vi "Write handle.vi"(8 "error in (no error)":errorcluster, 10 "handle":u64, 11 "Synnax Writer in":refnum<class "Synnax Writer.lvclass">) -> (0 "error out":errorcluster, 3 "Synnax Writer out":refnum<class "Synnax Writer.lvclass">)   [LabVIEW 2026, in "synnax_clib.lvlib" / "Synnax Writer.lvclass"]
uses:
  Synnax Writer.lvclass
  Synnax Writer.lvclass/Synnax Writer.ctl
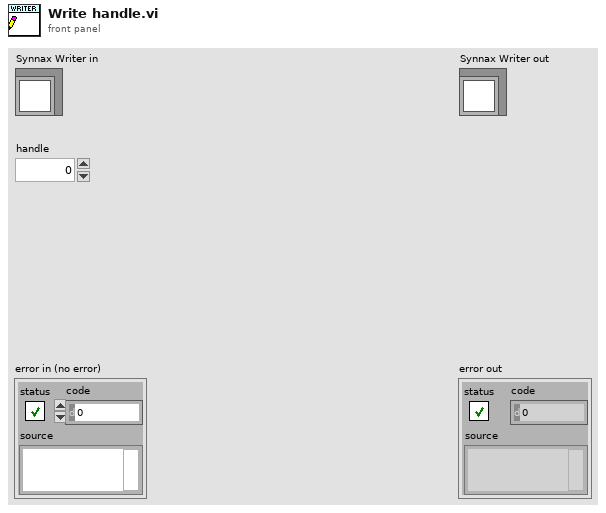
[diagram p1: front panel]
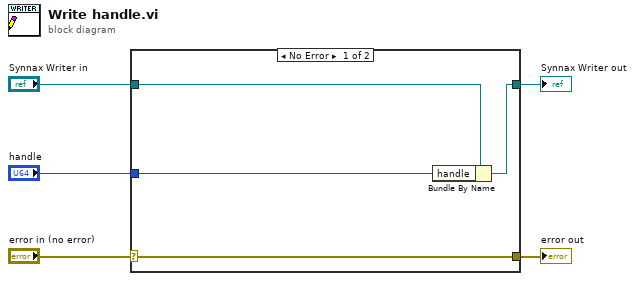
[diagram p0: block diagram]
diagram:
  n1 = case shown="No Error" "error in (no error)" {
    selector: "error in (no error)" -> [w9 w10]
    tunnel: [w9 w10] -> w4
    tunnel: [w7 w11] -> w2
    tunnel: "Synnax Writer in" -> [w8 w11]
    tunnel: "handle" -> [w6 _]
    frame No Error {
      n2 = Bundle By Name(cluster=w8, "handle"=w6) -> (w7:refnum<class "Synnax Writer.lvclass">)
    }
    frame Error {
    }
  }
  "error out" <- w4
  "Synnax Writer out" <- w2
